vi "UI Loop.vi"(4 "Loop":enum16{"Do Nothing", "Loop", "Stop"}(ring)) -> (1 "Loop Out":bool)   [LabVIEW 2009]
doc: "[Ver 1.00]\nREUSEABLE COMPONENT \nDESCRIPTION \nControls the loops within a multi-threaded system. Wire directly onto the condition of the While Loop. Use instead of global variables\n\nCOMMAND\nDo Nothing : Default Condition, returns whatever is set locally\nLoop : Outputs and sets a True\nStop : Outputs and sets a False \n\nERROR HANDLING\nNone\n------------------------------------------------------------------ \nVERSION CONTROL \nVer 1.00"
panel:
  # "Input"
  # "Output"
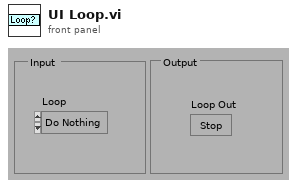
[diagram p1: front panel]
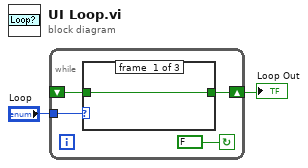
[diagram p0: block diagram]
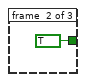
[diagram p2: hidden frame]
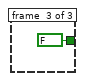
[diagram p3: hidden frame]
diagram:
  n1 = while {
    tunnel: "Loop" -> [w6]
    shift-left: _ -> [w4]
    shift-right: [w5] -> w1
    stop <- FALSE continue-if-true
    n2 = case shown="\"Loop\"" w6 {
      tunnel: [w7 TRUE FALSE] -> w5
      tunnel: w4 -> [w7 _ _]
      frame #0 {
      }
      frame #1 {
      }
      frame #2 {
      }
    }
  }
  "Loop Out" <- w1
